vi "termination.vi"(8 "Error In":errorcluster, 11 "GenAlg_data":T1) -> (0 "Error Out":errorcluster, 3 "GenAlg_data-out":T1, 4 "Stop":bool)   [LabVIEW 2016]
uses:
  TypeDefs/GenAlg_data.ctl
  TypeDefs/basic_config.ctl
  TypeDefs/element.ctl
  TypeDefs/geration_data.ctl
  TypeDefs/selection_data.ctl
  TypeDefs/SimulatedAnnealing_data.ctl
  TypeDefs/multi_eval_data.ctl
  TypeDefs/termination_data.ctl
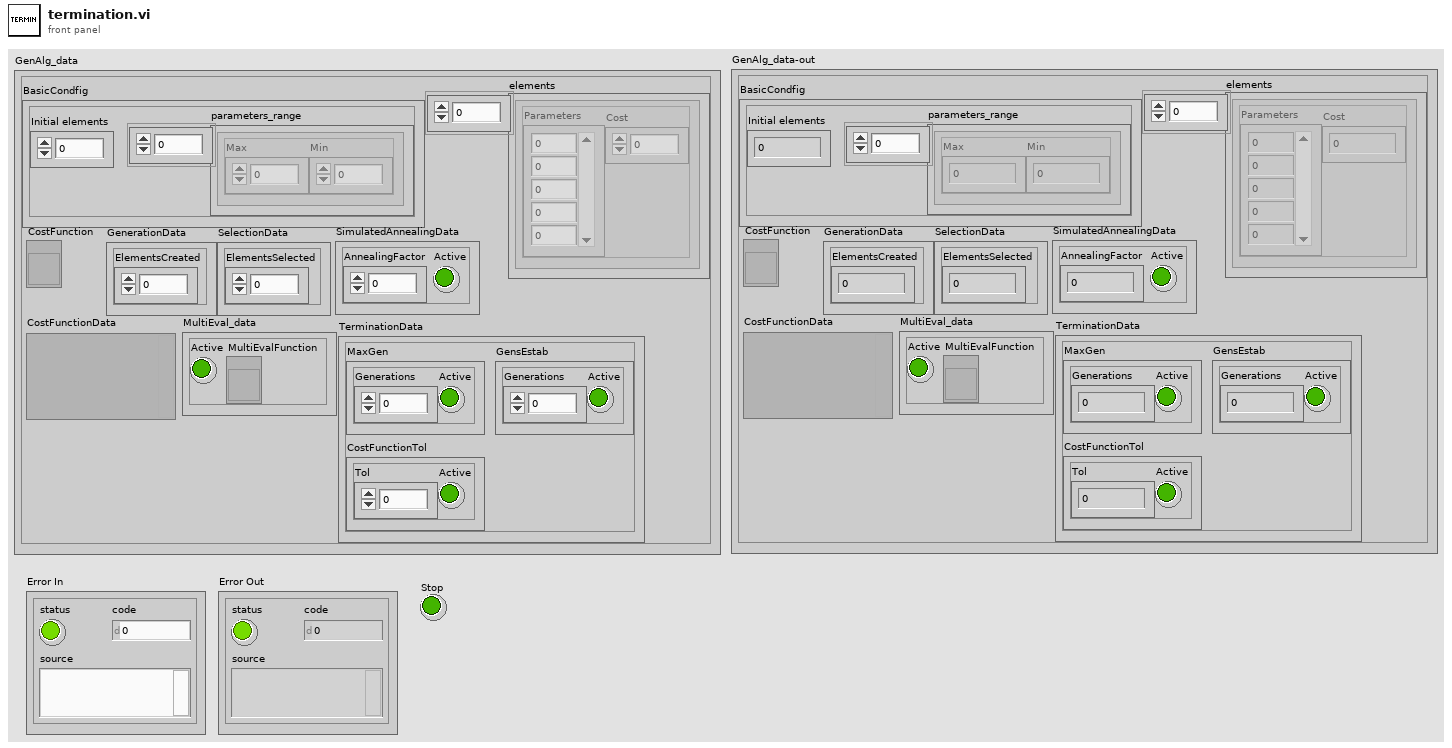
[diagram p1: front panel]
types:
  T1 = typedef "GenAlg_data.ctl" = cluster{"BasicCondfig":T2, "elements":T3[], "CostFunction":refnum<vi>, "GenerationData":T4, "SelectionData":T5, "SimulatedAnnealingData":T6, "CostFunctionData":variant, "MultiEval_data":T7, "TerminationData":T8}
  T2 = typedef "basic_config.ctl" = cluster{"parameters_range":cluster{"Max":dbl, "Min":dbl}[], "Initial elements":i32}
  T3 = typedef "element.ctl" = cluster{"Parameters":dbl[], "Cost":dbl}
  T4 = typedef "geration_data.ctl" = cluster{"ElementsCreated":i32}
  T5 = typedef "selection_data.ctl" = cluster{"ElementsSelected":i32}
  T6 = typedef "SimulatedAnnealing_data.ctl" = cluster{"AnnealingFactor":dbl, "Active":bool}
  T7 = typedef "multi_eval_data.ctl" = cluster{"Active":bool, "MultiEvalFunction":refnum<vi>}
  T8 = typedef "termination_data.ctl" = cluster{"MaxGen":cluster{"Generations":i32, "Active":bool}, "CostFunctionTol":cluster{"Tol":dbl, "Active":bool}, "GensEstab":cluster{"Generations":i32, "Active":bool}}
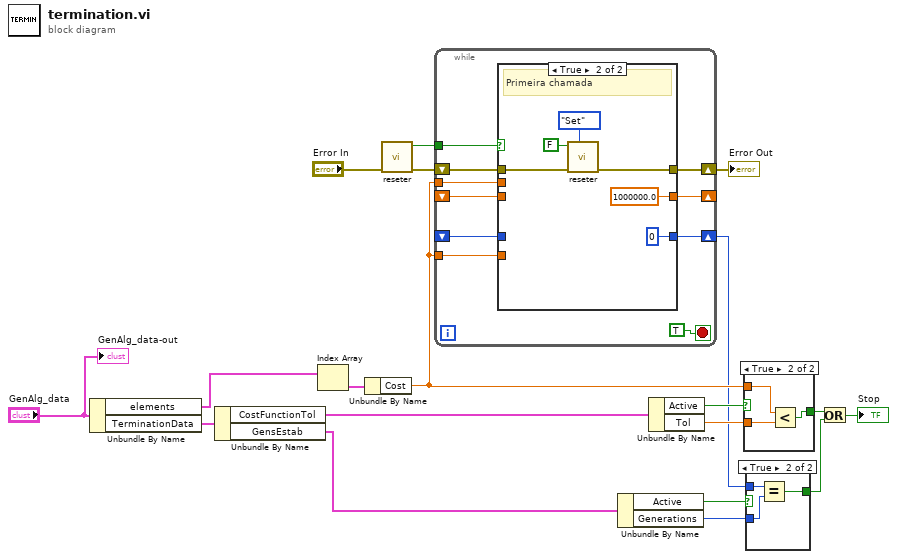
[diagram p0: block diagram]
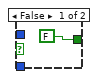
[diagram p2: hidden frame]
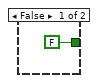
[diagram p3: hidden frame]
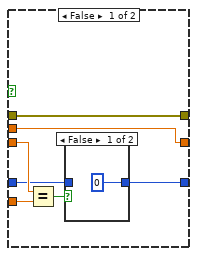
[diagram p4: hidden frame]
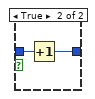
[diagram p5: hidden frame]
diagram:
  n1 = Unbundle By Name("GenAlg_data") -> ("elements"=w19:T3[], "TerminationData"=w16:T8)
  n2 = Unbundle By Name(w16) -> ("CostFunctionTol"=w15:cluster{"Tol":dbl, "Active":bool}, "GensEstab"=w9:cluster{"Generations":i32, "Active":bool})
  n3 = Index Array(array=w19) -> (element=w17:T3)  [unwired: 1 in]
  n4 = Unbundle By Name(w17) -> ("Cost"=w13:dbl)
  n5 = call "reseter.vi"("Error In"="Error In") -> ("Error Out"=w3:errorcluster, "Value"=w2:bool)  [unwired: 9 in]
  n6 = while {
    shift-right: [w29] -> w8
    shift-left: _ -> [w23]
    shift-right: [w28] -> _
    shift-left: _ -> [w25]
    tunnel: w13 -> [w26]
    tunnel: w13 -> [w24]
    shift-right: [w20] -> w1
    shift-left: w3 -> [w21]
    tunnel: w2 -> [w22]
    stop <- TRUE stop-if-true
    n7 = case shown="True" w22 {
      tunnel: [w31 0] -> w29
      tunnel: [w36 1000000.0] -> w28
      tunnel: w26 -> [w36 _]
      tunnel: w25 -> [w35 _]
      tunnel: w24 -> [w34 _]
      tunnel: w23 -> [w32 _]
      tunnel: w21 -> [w30 w43]
      tunnel: [w30 w42] -> w20
      frame False {
        n8 = Equal?(x=w35, y=w34) -> (x = y?=w33:bool)
        n9 = case shown="False" w33 {
          tunnel: w32 -> [_ w39]
          tunnel: [0 w38] -> w31
          frame False {
          }
          frame True {
            n10 = Increment(x=w39) -> (x+1=w38:i32)
          }
        }
      }
      frame True {
        # "Primeira chamada"
        n11 = call "reseter.vi"("Mode"=enum16{"Init", "Set", "Get"}."Set", "Error In"=w43, "Value"=FALSE) -> ("Error Out"=w42:errorcluster)  [unwired: 7 in, 1 out]
      }
    }
  }
  "Error Out" <- w1
  n12 = Unbundle By Name(w9) -> ("Active"=w10:bool, "Generations"=w11:i32)
  n13 = Unbundle By Name(w15) -> ("Active"=w14:bool, "Tol"=w12:dbl)
  n14 = case shown="True" w14 {
    tunnel: w13 -> [_ w49]
    tunnel: w12 -> [_ w48]
    tunnel: [FALSE w47] -> w6
    frame False {
    }
    frame True {
      n15 = Less?(x=w49, y=w48) -> (x < y?=w47:bool)
    }
  }
  n16 = case shown="True" w10 {
    tunnel: w8 -> [_ w53]
    tunnel: w11 -> [_ w52]
    tunnel: [FALSE w51] -> w7
    frame False {
    }
    frame True {
      n17 = Equal?(x=w53, y=w52) -> (x = y?=w51:bool)
    }
  }
  n18 = Or(x=w6, y=w7) -> (x .or. y?=→"Stop":bool)
  "GenAlg_data-out" <- "GenAlg_data"
